vi "PID Motor A.vi"(6 "PID gains":T2={"proportional gain (Kc)"=0.05, "integral time (Ti, min)"=0.003, "derivative time (Td, min)"=0.0} {"derivative time (Td, min)" format="%.6f"; "integral time (Ti, min)" format="%.6f"; "proportional gain (Kc)" format="%.6f"}, 7 "reinitialize? (F)":bool, 8 "error in (no error)":errorcluster, 9 "input":dbl, 10 "dt in (ms)":i32=-1, 11 "Setpoint A0":dbl(slide)=-0.016713091922005565 scale=-2.0..2.0) -> (0 "error out":errorcluster, 1 "dx/dt processed":dbl, 2 "output":dbl format="%.2f", 3 "Speed A0":T1(graph), 4 "dt out (s)":dbl format="%.3f", 5 "Counter A0":dbl)   [LabVIEW 2017]
uses:
  <vilib>/myRIO/Instrument Drivers/Onboard IO/PWM/typedefs/PWM Reference.ctl
  <vilib>/myRIO/Common/Instrument Driver Framework/Utilities/typedefs/myRIO Generic Hardware Reference.ctl
  <vilib>/myRIO/Common/Instrument Driver Framework/Utilities/typedefs/Hardware Version Enum.ctl
  <vilib>/myRIO/Common/Instrument Driver Framework/Utilities/typedefs/myRIO v1.0 Reference.ctl
  <vilib>/myRIO/Common/Instrument Driver Framework/Utilities/typedefs/Generic FPGA Reference.ctl
  <vilib>/myRIO/Common/Instrument Driver Framework/myRIO v1.0/PWM/typedefs/PWM Channels Enum.ctl
  <vilib>/myRIO/Instrument Drivers/Onboard IO/PWM/typedefs/PWM Configuration.ctl
  <vilib>/userdefined/High Color/nirio_resource_hc.ctl
  <vilib>/myRIO/Common/Instrument Driver Framework/Utilities/vis/Is FPGA Ref Available.vi
  <vilib>/myRIO/Common/Instrument Driver Framework/myRIO v1.0/PWM/vis/myRIO v1.1 Open PWM.vi
  <vilib>/myRIO/Instrument Drivers/Onboard IO/PWM/vis/Set Duty Cycle and Frequency.vi
  <vilib>/myRIO/Common/Instrument Driver Framework/Utilities/vis/Validate Channels.vi
  <vilib>/myRIO/Common/Instrument Driver Framework/myRIO v1.0/PWM/vis/myRIO v1.0 Reserve PWM.vi
  <vilib>/myRIO/Common/Instrument Driver Framework/myRIO v1.0/PWM/vis/myRIO v1.0 Build MUX Configuration PWM.vi
  <vilib>/myRIO/Common/Instrument Driver Framework/myRIO v1.0/Resource Manager/vis/myRIO v1.0 Reserve Channel List.vi
  <vilib>/myRIO/Common/Instrument Driver Framework/myRIO v1.0/Resource Manager/vis/myRIO v1.0 Create Configuration List.vi
  <vilib>/myRIO/Common/Instrument Driver Framework/myRIO v1.0/Resource Manager/vis/myRIO v1.0 Reserve Channel.vi
  <vilib>/myRIO/Common/Instrument Driver Framework/myRIO v1.0/Resource Manager/vis/myRIO v1.0 Unreserve Channel.vi
  <vilib>/myRIO/Common/Instrument Driver Framework/myRIO v1.0/Resource Manager/vis/myRIO v1.0 Build Mutex Name.vi
  <vilib>/Utility/VariantDataType/GetNumericInfo.vi
  <vilib>/Utility/error.llb/Error Cluster From Error Code.vi
  <vilib>/myRIO/Common/Instrument Driver Framework/myRIO v1.0/myRIO v1.1 Open.vi
  <vilib>/myRIO/Common/Instrument Driver Framework/Utilities/vis/IO Manager.vi
  <vilib>/myRIO/Common/Instrument Driver Framework/Utilities/vis/Configuration Manager.vi
  <vilib>/myRIO/Common/Instrument Driver Framework/myRIO v1.0/Resource Manager/vis/myRIO v1.0 Configure IO.vi
  <vilib>/myRIO/Common/Instrument Driver Framework/myRIO v1.0/myRIO v1.0 Close.vi
  <vilib>/myRIO/Common/Instrument Driver Framework/myRIO v1.0/PWM/vis/myRIO v1.0 Write PWM.vi
  <vilib>/addons/control/pid/pid.llb/PID (DBL).vi
  <vilib>/myRIO/Express VI/Onboard IO/PWM/PWM Express VI.xnode
  <vilib>/myRIO/Instrument Drivers/Onboard IO/PWM/vis/myRIO PWM Open.xnode
  <vilib>/myRIO/Instrument Drivers/Onboard IO/PWM/PWM.lvlib
  <vilib>/addons/control/pid/NI_PID_pid.lvlib
panel:
  in  "Encoder accuracy multiplier":dbl=0.926
  in  "Adjust speed multiplier":dbl=1.0
  out "dx/dt measured":dbl
  out "Setpoint":dbl
  # "VI Description: Converts the input into a PWM value to move the motor, measures the velocity of a motor,\nthen recalculates the new input (in the form of the output)"
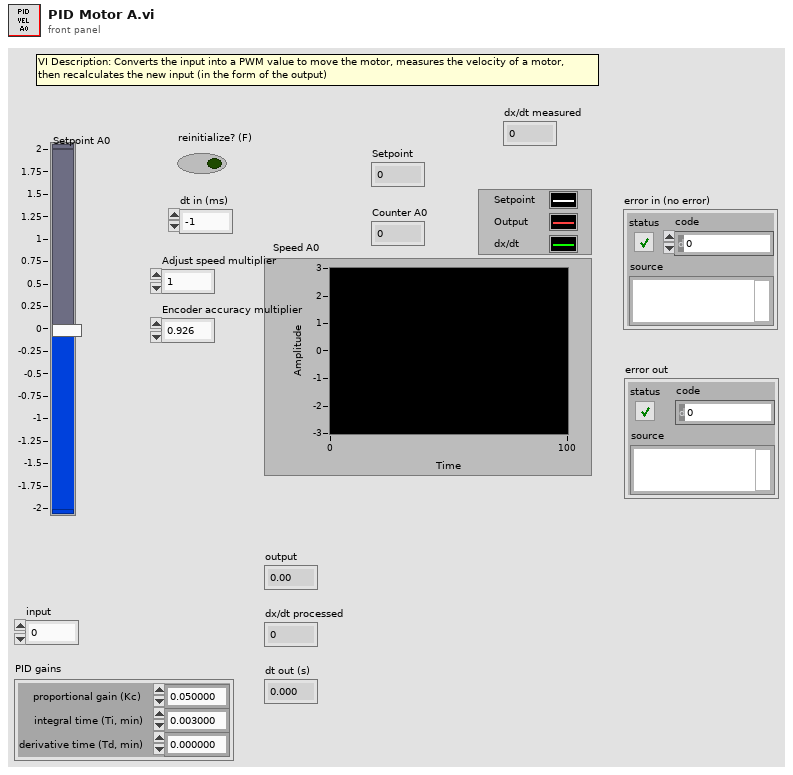
[diagram p1: front panel]
types:
  T1 = cluster{"Setpoint":dbl, "output":dbl, "dx/dt":dbl}
  T2 = cluster{"proportional gain (Kc)":dbl, "integral time (Ti, min)":dbl, "derivative time (Td, min)":dbl}
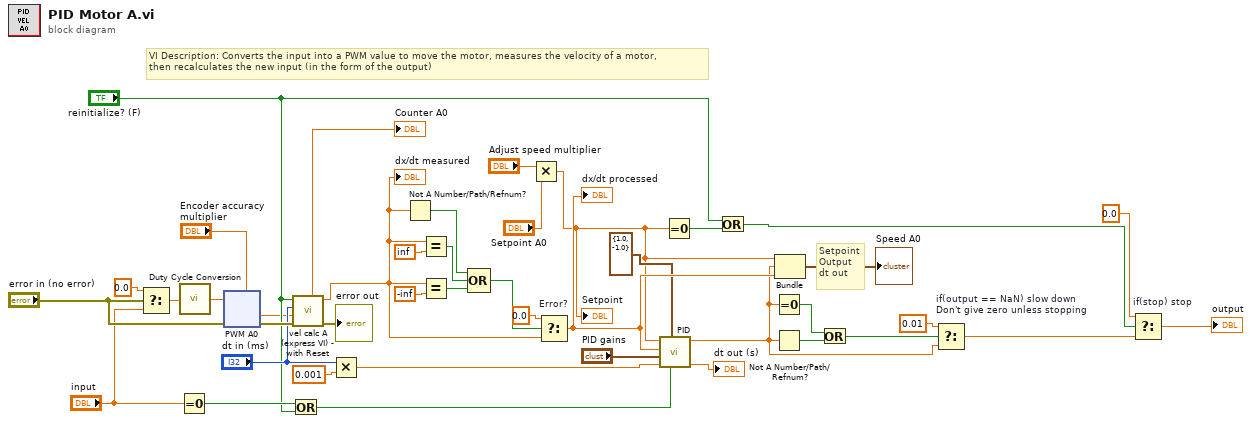
[diagram p0: block diagram]
diagram:
  # "VI Description: Converts the input into a PWM value to move the motor, measures the velocity of a motor,\nthen recalculates the new input (in the form of the output)"
  # "Setpoint\nOutput\ndt out"
  n1 = Select(t=0.0, s="error in (no error)", f="input") -> (s? t:f=w5:dbl)
  n2 = Equal To 0?(x="input") -> (x = 0?=w11:bool)
  n3 = call "Duty Cycle Conversion.vi"("Duty Cycle In"=w5) -> ("Duty Cyle Out"=w34:dbl)
  n4 = xnode "PWM A0"("error in (no error)"="error in (no error)", "Duty Cycle"=w34) -> ("error out"=w33:errorcluster)
  n5 = Or(x=w11, y="reinitialize? (F)") -> (x .or. y?=w9:bool)
  n6 = call "vel calc A (express VI) - with Reset.vi"("error in"=w33, "Encoder accuracy multiplier"="Encoder accuracy multiplier", "dt in (ms)"="dt in (ms)", "Reinitialise"="reinitialize? (F)") -> ("error out"=→"error out":errorcluster, "dx/dt"=w22:dbl, "Counter Value"=→"Counter A0":dbl)  [unwired: 3 in, 2 out]
  "dx/dt measured" <- w22
  n7 = Multiply(x="dt in (ms)", y=0.001) -> (x*y=w30:dbl)
  n8 = Not A Number/Path/Refnum?(number/path/refnum=w22) -> (NaN/Path/Refnum?=w24:bool)
  n9 = Equal?(x=w22, y=inf) -> (x = y?=w25:bool)
  n10 = Equal?(x=w22, y=-inf) -> (x = y?=w26:bool)
  n11 = Compound Arithmetic op=OR(w24, w25, w26) -> (w23:bool)
  n12 = Multiply(x="Adjust speed multiplier", y="Setpoint A0") -> (x*y=w2:dbl)
  "Setpoint" <- w2
  n13 = Select "Error?"(t=0.0, s=w23, f=w22) -> (s? t:f=w41:dbl)
  "dx/dt processed" <- w41
  n14 = call-poly <vilib>:"PID.vi"("reinitialize? (F)"=w9, "output range"=cluster{"output high":dbl, "output low":dbl} {"output high"=1.0, "output low"=-1.0}, "dt (s)"=w30, "PID gains"="PID gains", "process variable"=w41, "setpoint"=w2) -> ("dt out (s)"=→"dt out (s)":dbl, "output"=w17:dbl)  [unwired: 4 in]
  n15 = Equal To 0?(x=w2) -> (x = 0?=w13:bool)
  n16 = Or(x="reinitialize? (F)", y=w13) -> (x .or. y?=w12:bool)
  n17 = Equal To 0?(x=w17) -> (x = 0?=w16:bool)
  n18 = Not A Number/Path/Refnum?(number/path/refnum=w17) -> (NaN/Path/Refnum?=w15:bool)
  n19 = Bundle(w2, "output"=w17, "dx/dt"=w41) -> (→"Speed A0":cluster{dbl, "output":dbl, "dx/dt":dbl})  [unwired: 1 in]
  n20 = Or(x=w16, y=w15) -> (x .or. y?=w14:bool)
  n21 = Select "if(output == NaN) slow down\nDon't give zero unless stopping"(t=0.01, s=w14, f=w17) -> (s? t:f=w20:dbl)
  n22 = Select "if(stop) stop"(t=0.0, s=w12, f=w20) -> (s? t:f=→"output":dbl)
